vi "Write XtraJsonEncodeObj.vi"(8 "error in (no error)":errorcluster, 10 "XtraJsonEncodeObj":bool, 11 "LogMap in":refnum<class "LogMap.lvclass">) -> (0 "error out":errorcluster, 3 "LogMap out":refnum<class "LogMap.lvclass">)   [LabVIEW 2020, in "ORM.lvlib" / "LogMap.lvclass"]
uses:
  LogMap.lvclass
  LogMap.lvclass/LogMap.ctl
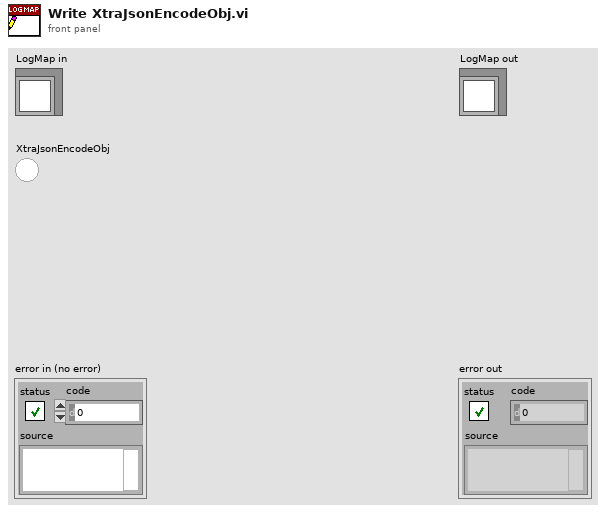
[diagram p1: front panel]
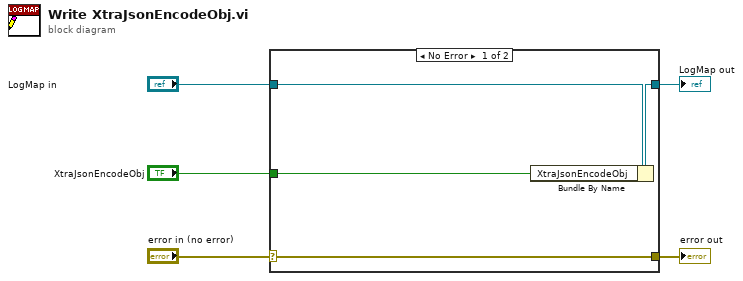
[diagram p0: block diagram]
diagram:
  n1 = case shown="No Error" "error in (no error)" {
    selector: "error in (no error)" -> [w9 w10]
    tunnel: [w9 w10] -> w4
    tunnel: [w7 w11] -> w2
    tunnel: "LogMap in" -> [w8 w11]
    tunnel: "XtraJsonEncodeObj" -> [w6 _]
    frame No Error {
      n2 = Bundle By Name(cluster=w8, "XtraJsonEncodeObj"=w6) -> (w7:refnum<class "LogMap.lvclass">)
    }
    frame Error {
    }
  }
  "error out" <- w4
  "LogMap out" <- w2
